vi "submove.vi"(8 "error in (no error)":errorcluster, 9 "error in (no error) 2":errorcluster, 10 "Wavelength":dbl=795.0, 11 "reference":refnum<k7>) -> (1 "Wavelength 2":dbl, 2 "Angle":dbl, 3 "x < 0?":bool)   [LabVIEW 2019]
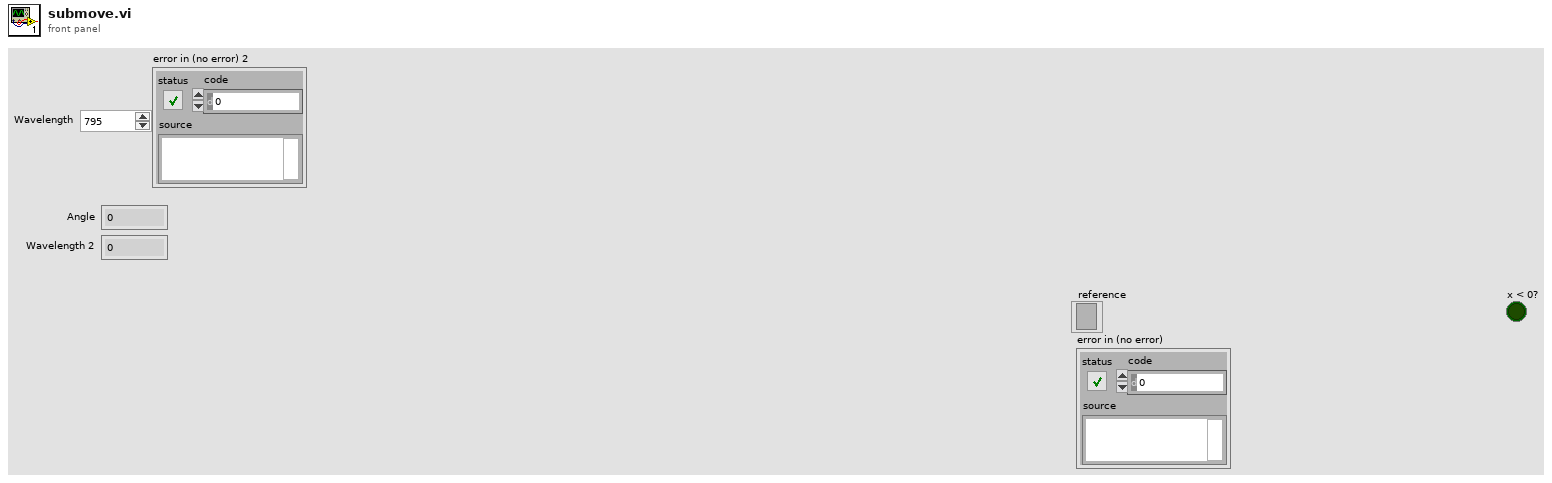
[diagram p1: front panel]
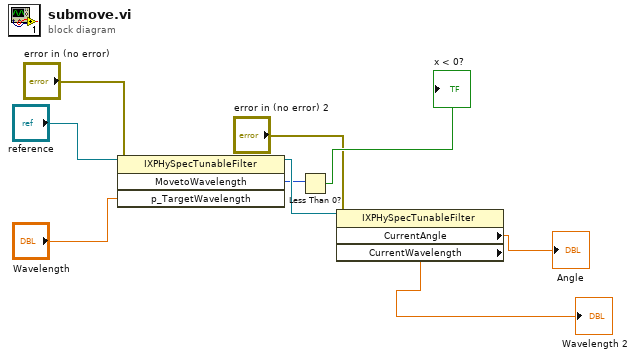
[diagram p0: block diagram]
diagram:
  n1 = invoke class="IXPHySpecTunableFilter" method="MovetoWavelength"(reference="reference", error in="error in (no error)", "p_TargetWavelength"="Wavelength") -> (reference out=w7:refnum<k7>, "MovetoWavelength"=w5:i32)  [unwired: 1 in, 2 out]
  n2 = Less Than 0?(x=w5) -> (x < 0?=→"x < 0?":bool)
  n3 = property class="IXPHySpecTunableFilter"(reference=w7, error in="error in (no error) 2") -> ("CurrentAngle"=→"Angle":dbl, "CurrentWavelength"=→"Wavelength 2":dbl)  [unwired: 2 out]
